vi "SV Time-Varying Loudness (Intensity_2014).vi"(0 "sound pressure signal [Pa]":waveform(dbl)={"t0"=timestamp(0 s since 1904-01-01), "dt"=0.0, "Y"=[]}, 1 "diffuse field":bool, 2 "reset":bool, 11 "error in (no error)":errorcluster) -> (4 "specific loudness [Sones/Bark]":dbl[][](array[numeric]), 6 "time-varying loudness [Sones]":waveform(dbl), 8 "offset and multipliers":T1={"t0 and delta t [s]"={"t0"=0.0, "delta t"=0.0}, "y0 and delta y [Bark]"={"y0"=0.0, "delta y"=0.0009765625}} {"y0 and delta y [Bark]"."delta y" format="%.2f"; "y0 and delta y [Bark]"."y0" format="%.2f"; "t0 and delta t [s]"."delta t" format="%.2f"; "t0 and delta t [s]"."t0" format="%.2f"}, 10 "loudness info":T2, 15 "error out":errorcluster)   [LabVIEW 2017, in "SoundVib_SoundQuality.lvlib"]
doc: "Computes time-varying loudness of the sound pressure signal from a time-varying 1/3 octave band spectrum."
uses:
  <vilib>/addons/Sound and Vibration/svt_Sound Quality/SoundVib_SoundQuality.lvlib
  <vilib>/addons/_NISVFA/_Shared subVIs/Controls/svc_SQ Info.ctl
  <vilib>/addons/_NISVFA/_Shared subVIs/Common/SVL Set dB Reference (1 Ch).vi
  <vilib>/addons/_NISVFA/_Shared subVIs/Common/SVL Set dB Reference (variant).vi
  <vilib>/addons/_NISVFA/_Shared subVIs/Common/svc_Get Array Subset (Index).vi
  <vilib>/addons/_NISVFA/_Shared subVIs/Common/svc_Coerce Index and Length.vi
  <vilib>/addons/_NISVFA/_Shared subVIs/Common/svc_Conditional Merge Error.vi
  <vilib>/addons/Sound and Vibration/svt_Octave_2014 standard/SVT Third-octave Analysis (1 Ch).vi
  <vilib>/addons/_NISVFA/_Shared subVIs/Common/svc_Caller VI Returned in Error Source.vi
  <vilib>/Waveform/WDTOps.llb/WDT Append Waveforms DBL.vi
  <vilib>/addons/Sound and Vibration/svt_Octave/SoundVib_Octave_2014 standard.lvlib
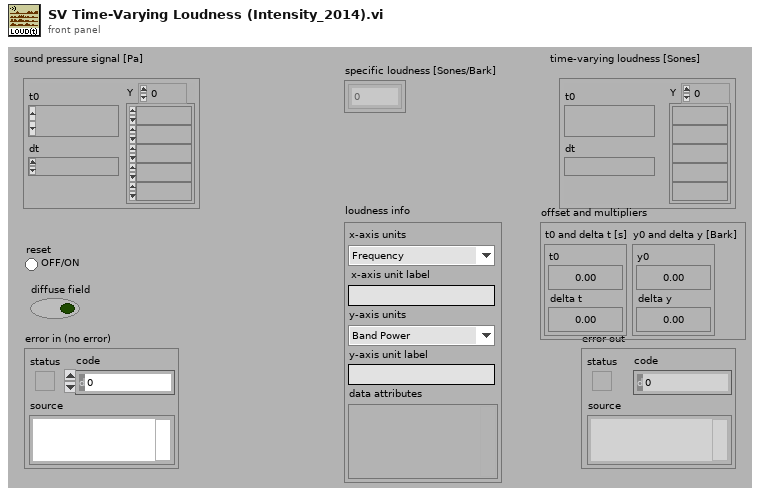
[diagram p1: front panel]
types:
  T1 = cluster{"t0 and delta t [s]":cluster{"t0":dbl, "delta t":dbl}, "y0 and delta y [Bark]":cluster{"y0":dbl, "delta y":dbl}}
  T2 = typedef "svc_SQ Info.ctl" = cluster{"x-axis units":enum16{"Frequency", "Critical Band", "Critical Band Rate"}, "x-axis unit label":string, "y-axis units":enum16{"Band Power", "Level", "Loudness", "Sharpness", "Roughness", "Fluctuation Strength", "Tonality"}, "y-axis unit label":string, "data attributes":variant}
  T3 = cluster{"mode":enum16{"Slow", "Fast", "Impulse", "Custom"}, "time constant [ms]":dbl}
  T4 = enum16{"Linear", "Exponential", "Equal confidence", "Peak"}
  T5 = cluster{"low band":enum16{"20 Hz", "25 Hz", "31.5 Hz", "40 Hz", "50 Hz", "63 Hz", "80 Hz", "100 Hz", "125 Hz", "160 Hz", "200 Hz", "250 Hz", "315 Hz", "400 Hz", "500 Hz", "630 Hz", "800 Hz", "1000 Hz", "1250 Hz", "1600 Hz", "2000 Hz", "2500 Hz", "3150 Hz", "4000 Hz", "5000 Hz", "6300 Hz", "8000 Hz", "10000 Hz", "12500 Hz", "16000 Hz", "20000 Hz"}, "high band":enum16{"20 Hz", "25 Hz", "31.5 Hz", "40 Hz", "50 Hz", "63 Hz", "80 Hz", "100 Hz", "125 Hz", "160 Hz", "200 Hz", "250 Hz", "315 Hz", "400 Hz", "500 Hz", "630 Hz", "800 Hz", "1000 Hz", "1250 Hz", "1600 Hz", "2000 Hz", "2500 Hz", "3150 Hz", "4000 Hz", "5000 Hz", "6300 Hz", "8000 Hz", "10000 Hz", "12500 Hz", "16000 Hz", "20000 Hz"}}
  T6 = enum16{"Linear", "Linear + Bark edges", "Critical-band rates", "Critical band centers"}
  T7 = cluster{"nominal frequencies [Hz]":dbl[], "band power":dbl[]}
  T8 = cluster{"resolution (Bark)":dbl, "resolution (Bark)":dbl}
  T9 = cluster{cluster{dbl, dbl}, cluster{"resolution (Bark)":dbl, "resolution (Bark)":dbl}}
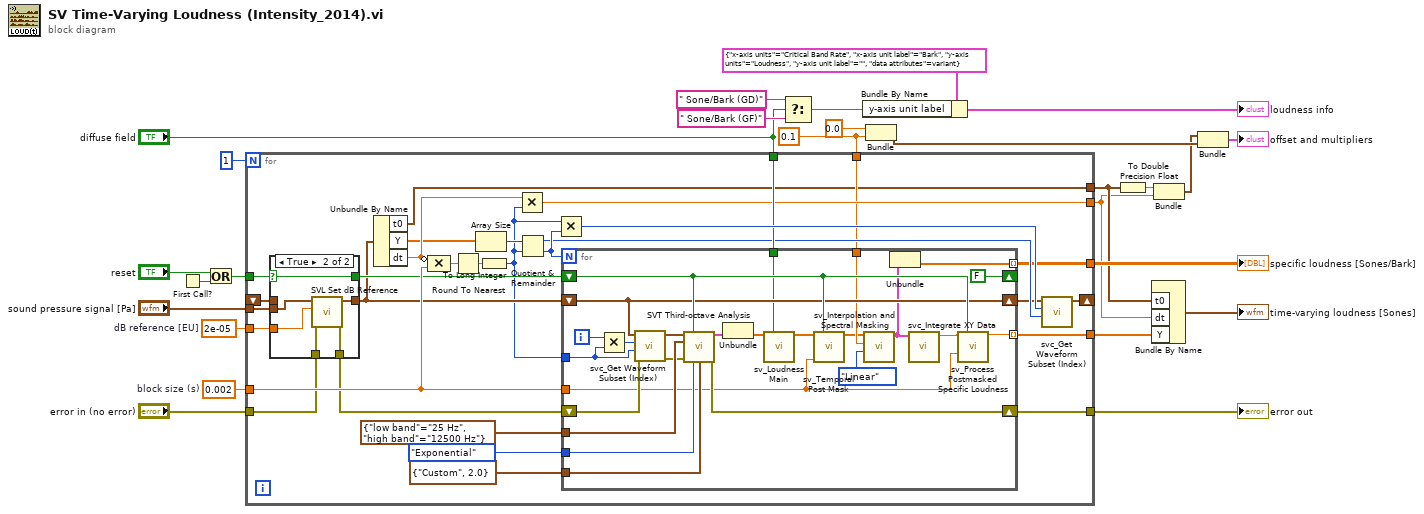
[diagram p0: block diagram]
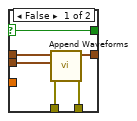
[diagram p2: hidden frame]
diagram:
  w1 = 2e-05  # dB reference [EU]
  w5 = 0.1 ("resolution (Bark)")
  w21 = 0.002  # block size (s)
  n1 = First Call?() -> (First Call?: T/F=w26:bool)
  n2 = Or(x="reset", y=w26) -> (x .or. y?=w23:bool)
  n3 = for {
    N: 1 -> [_]
    tunnel: w21 -> [w44]
    shift-right: [w54] -> _
    shift-left: _ -> [w56]
    tunnel: "sound pressure signal [Pa]" -> [w52]
    tunnel: w23 -> [w55]
    tunnel: "error in (no error)" -> [w34]
    tunnel: [w43] -> w19
    tunnel: "diffuse field" -> [w40]
    tunnel: [w32] -> w12
    tunnel: [w31] -> w11
    tunnel: [w27] -> w9
    tunnel: [w30] -> w7
    tunnel: w5 -> [w29]
    tunnel: w1 -> [w28]
    n4 = case shown="True" w55 {
      selector: w55 -> [w84 w93]
      tunnel: w56 -> [w86 _]
      tunnel: w52 -> [w87 w92]
      tunnel: [w85 w91] -> w37
      tunnel: [w84 w93] -> w42
      tunnel: w34 -> [w83 w90]
      tunnel: [w82 w89] -> w33
      tunnel: w28 -> [_ w88]
      frame False {
        n5 = call-poly <vilib>:"Append Waveforms.vi"("error in (no error)"=w83, "waveform B"=w87, "waveform A"=w86) -> ("error out"=w82:errorcluster, "waveform out"=w85:waveform(dbl))  [unwired: 7 in]
      }
      frame True {
        n6 = call-poly <vilib>:"SVL Set dB Reference.vi"("error in (no error)"=w90, "dB reference [EU]"=w88, "scaled signal in [EU]"=w92) -> ("error out"=w89:errorcluster, "scaled signal out [EU]"=w91:waveform(dbl))  [unwired: 7 in]
      }
    }
    n7 = Unbundle By Name(w37) -> ("t0"=w27:timestamp, "Y"=w36:dbl[], "dt"=w41:dbl)
    n8 = Compound Arithmetic op=MULTIPLY(invert w41, w44) -> (w50:dbl)
    n9 = Round To Nearest(number=w50) -> (nearest integer value=w49:dbl)
    n10 = Array Size(array=w36) -> (size(s)=w51:i32)
    n11 = To Long Integer(number=w49) -> (32bit integer=w35:i32)
    n12 = Multiply(x=w41, y=w35) -> (x*y=w30:dbl)
    n13 = Quotient & Remainder(x=w51, y=w35) -> (x-y*floor(x/y)=w39:i32, floor(x/y)=w48:i32)
    n14 = Multiply(x=w35, y=w48) -> (x*y=w53:i32)
    n15 = for {
      N: w48 -> [_]
      tunnel: w35 -> [w79]
      tunnel: T5 {"low band"=enum."25 Hz", "high band"=enum."12500 Hz"} ("frequency range") -> [w77]
      tunnel: T4."Exponential" ("averaging type") -> [w75]
      tunnel: T3 {"mode"=enum."Custom", "time constant [ms]"=2.0} ("exp avg settings") -> [w74]
      tunnel: w44 -> [w65]
      shift-right: [w68] -> w43
      shift-left: w33 -> [w73]
      tunnel: [w72] -> w31 mode=indexing
      shift-right: [FALSE] -> _
      shift-left: w42 -> [w71]
      tunnel: w40 -> [w66]
      shift-right: [w69] -> w38
      shift-left: w37 -> [w69]
      tunnel: w29 -> [w64]
      tunnel: [w61] -> w32 mode=indexing
      i -> [w81]
      n16 = Multiply(x=w81, y=w79) -> (x*y=w80:i32)
      n17 = call <vilib>:"svc_Get Waveform Subset (Index).vi"("error in (no error)"=w73, "length (-1 = all)"=w79, "start index (0)"=w80, "waveform in"=w69) -> ("error out"=w76:errorcluster, "waveform subset"=w78:waveform(dbl))  [unwired: 2 in, 4 out]
      n18 = call-poly <vilib>:"SVT Third-octave Analysis.vi"("scaled signal [EU]"=w78, "restart averaging (F)"=w71, "frequency range"=w77, "error in (no error)"=w76, "averaging type"=w75, "exp avg settings"=w74) -> ("octave spectrum"=w67:T7, "error out"=w68:errorcluster)  [unwired: 4 in, 4 out]
      n19 = Unbundle(w67) -> ("band power"=w63:dbl[])  [unwired: 1 out]
      n20 = call <vilib>:"sv_Loudness Main.vi"("1/3 OB Spectrum"=w63, "Diffuse Field?"=w66) -> ("Main Loudness"=w60:dbl[])  [unwired: 13 in]
      n21 = call <vilib>:"sv_Temporal Post Mask.vi"("specific loudness"=w60, "restart"=w71, "dt"=w65) -> ("specific loudness"=w59:dbl[])  [unwired: 12 in]
      n22 = call <vilib>:"sv_Interpolation and Spectral Masking.vi"("interpolation type"=T6."Linear", "resolution (Bark)"=w64, "Nm"=w59) -> ("specifc loudness"=w58:cluster{"Bark (X)":dbl[], "Nm (Y)":dbl[]})  [unwired: 8 in]
      n23 = Unbundle(w58) -> ("Nm (Y)"=w61:dbl[])  [unwired: 1 out]
      n24 = call <vilib>:"svc_Integrate XY Data.vi"("XY"=w58) -> ("integral(ydx)"=w57:dbl)  [unwired: 10 in]
      n25 = call <vilib>:"sv_Process Postmasked Specific Loudness.vi"("total loudness N*(t)"=w57, "reset"=w71, "dt (s)"=w65) -> ("total loudness N(t)"=w72:dbl)  [unwired: 12 in]
    }
    n26 = call <vilib>:"svc_Get Waveform Subset (Index).vi"("length (-1 = all)"=w39, "start index (0)"=w53, "waveform in"=w38) -> ("waveform subset"=w54:waveform(dbl))  [unwired: 3 in, 5 out]
  }
  "specific loudness [Sones/Bark]" <- w12
  "error out" <- w19
  n27 = Select(t=" Sone/Bark (GD)", s="diffuse field", f=" Sone/Bark (GF)") -> (s? t:f=w15:string)
  n28 = Bundle By Name(cluster=T2 {"x-axis units"=enum."Critical Band Rate", "x-axis unit label"="Bark", "y-axis units"=enum."Loudness", "y-axis unit label"="", "data attributes"=variant} ("loudness info"), "y-axis unit label"=w15) -> (→"loudness info":T2)
  n29 = Bundle("resolution (Bark)"=0.0, "resolution (Bark)"=w5) -> (w3:T8)  [unwired: 1 in]
  n30 = To Double Precision Float(number=w9) -> (double precision float=w8:dbl)
  n31 = Bundle By Name("t0"=w9, "dt"=w7, "Y"=w11) -> (→"time-varying loudness [Sones]":waveform(dbl))  [unwired: 1 in]
  n32 = Bundle(w8, w7) -> (w2:cluster{dbl, dbl})  [unwired: 1 in]
  n33 = Bundle(w2, w3) -> (→"offset and multipliers":T9)  [unwired: 1 in]
